vi "Prova 1.vi"(0 "Integer":dbl, 5 "Boolean":bool) -> (4 "Numeric":dbl)   [LabVIEW 2021]
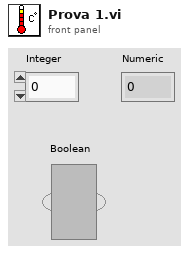
[diagram p1: front panel]
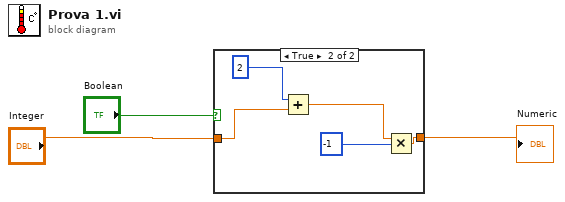
[diagram p0: block diagram]
diagram:
  n1 = case shown="True" "Boolean" {
    tunnel: [w4 w8] -> w3
    tunnel: "Integer" -> [w4 w5]
    frame False {
    }
    frame True {
      n2 = Add(x=2, y=w5) -> (x+y=w7:dbl)
      n3 = Multiply(x=w7, y=-1) -> (x*y=w8:dbl)
    }
  }
  "Numeric" <- w3
